vi "Convert to Array Data in Single Current Mode.vi"(7 "External\nRef":bool=TRUE, 8 "data":dbl[](array[numeric]), 9 "Electrode number, N":u16=8, 10 "Current Mode":u8[](array[numeric]), 11 "Array Mode":u16(ring) items=["None", "Gradient + Dipole dipole", "Gradient", "Dipole Dipole", "Schlumberger"]) -> (3 "String":string)   [LabVIEW 2023]
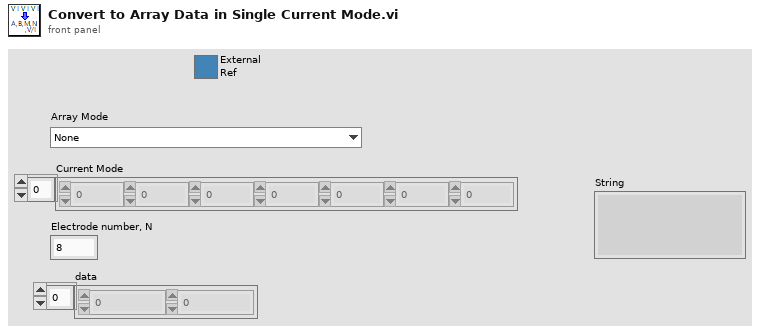
[diagram p1: front panel]
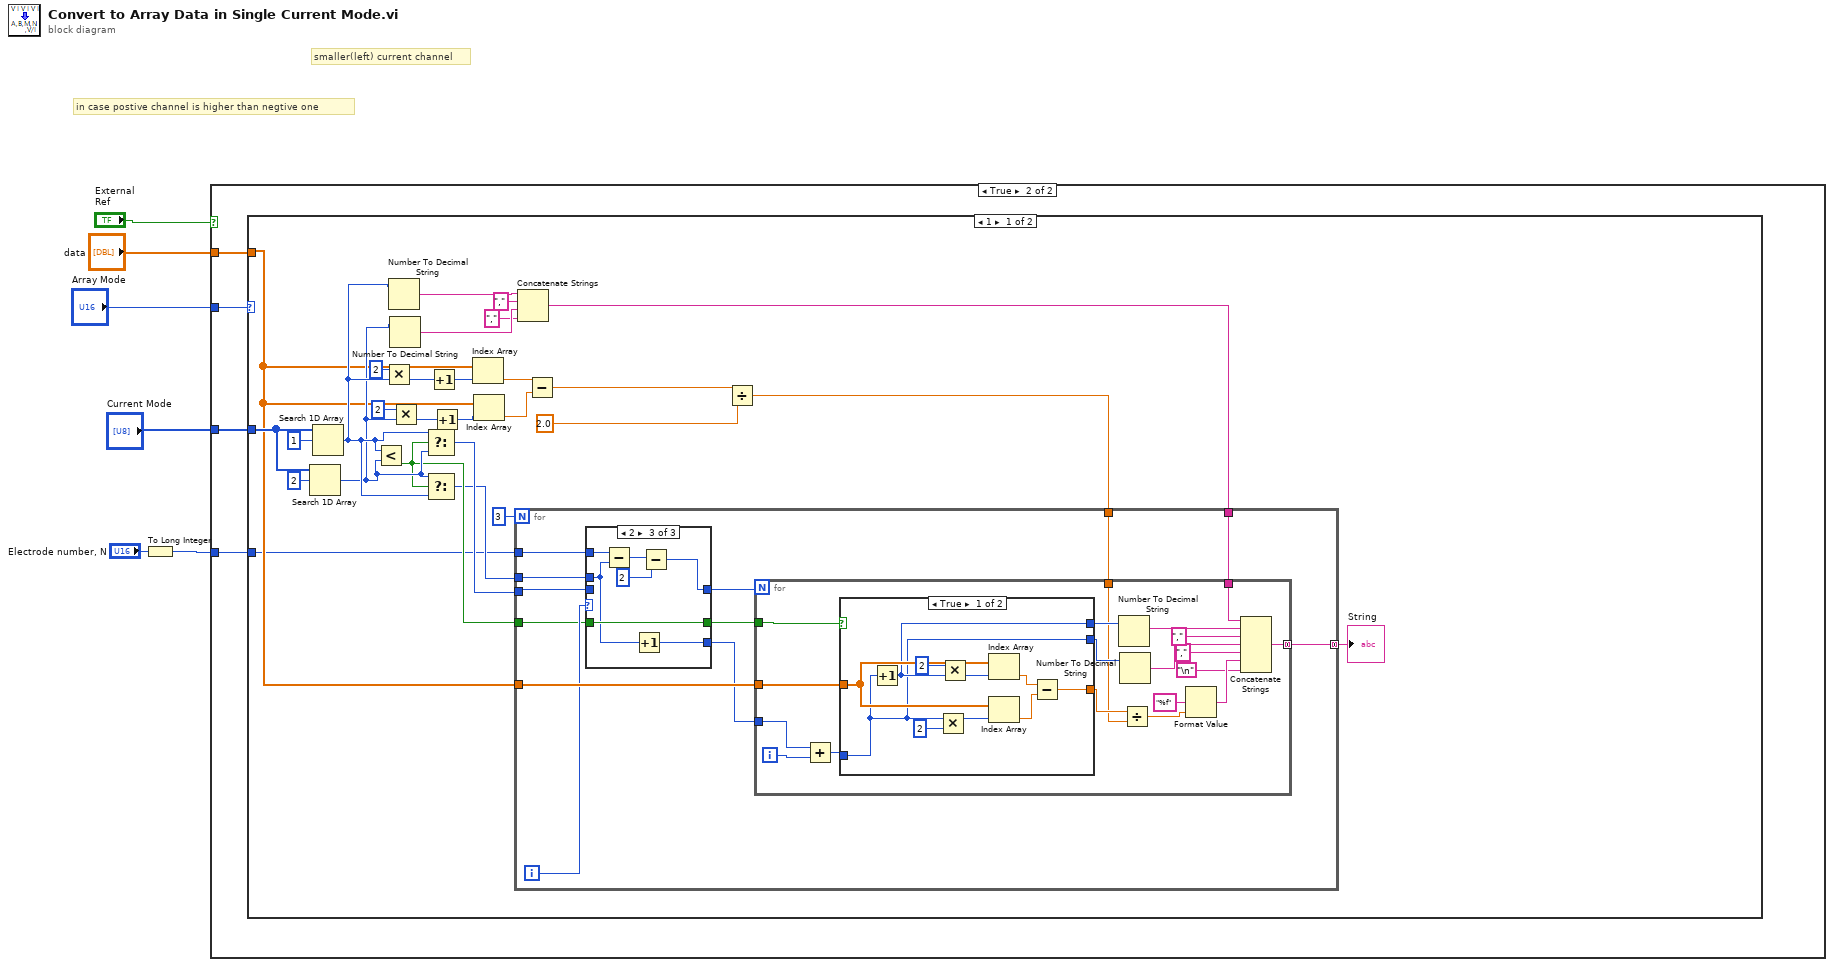
[diagram p0: block diagram]
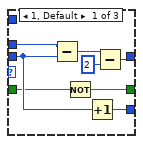
[diagram p3: hidden frame]
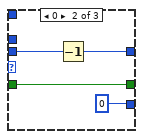
[diagram p4: hidden frame]
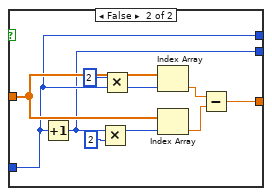
[diagram p5: hidden frame]
diagram:
  # "smaller(left) current channel"
  # "in case postive channel is higher than negtive one"
  n1 = To Long Integer(number="Electrode number, N") -> (32bit integer=w1:i32)
  n2 = case shown="True" "External\nRef" {
    tunnel: "Array Mode" -> [_ w10]
    tunnel: "Current Mode" -> [_ w9]
    tunnel: "data" -> [_ w8]
    tunnel: w1 -> [_ w7]
    frame False {
    }
    frame True {
      n3 = case shown="1" w10 {
        tunnel: w9 -> [w36 _]
        tunnel: w8 -> [w16 _]
        tunnel: w7 -> [w11 _]
        frame 1 {
          n4 = Search 1D Array(1D array=w36, element=u8 2) -> (index of element=w30:i32)  [unwired: 1 in]
          n5 = Search 1D Array(1D array=w36, element=u8 1) -> (index of element=w31:i32)  [unwired: 1 in]
          n6 = Less?(x=w31, y=w30) -> (x < y?=w19:bool)
          n7 = Multiply(x=2, y=w31) -> (x*y=w25:i32)
          n8 = Number To Decimal String(number=w31) -> (decimal integer string=w35:string)  [unwired: 1 in]
          n9 = Number To Decimal String(number=w30) -> (decimal integer string=w33:string)  [unwired: 1 in]
          n10 = Multiply(x=2, y=w30) -> (x*y=w22:i32)
          n11 = Select(t=w31, s=w19, f=w30) -> (s? t:f=w14:i32)
          n12 = Select(t=w30, s=w19, f=w31) -> (s? t:f=w13:i32)
          n13 = Increment(x=w25) -> (x+1=w23:i32)
          n14 = Increment(x=w22) -> (x+1=w20:i32)
          n15 = Index Array(array=w16, index=w23) -> (element=w29:dbl)
          n16 = Index Array(array=w16, index=w20) -> (element=w28:dbl)
          n17 = Concatenate Strings(w35, "," ("string"), w33, "," ("string")) -> (w17:string)
          n18 = Subtract(x=w29, y=w28) -> (x-y=w27:dbl)
          n19 = Divide(x=w27, y=2.0) -> (x/y=w18:dbl)
          n20 = for {
            N: 3 -> [_]
            tunnel: w19 -> [w44]
            tunnel: w18 -> [w50]
            tunnel: w17 -> [w49]
            tunnel: w16 -> [w48]
            tunnel: w14 -> [w47]
            tunnel: w13 -> [w41]
            tunnel: [w40] -> w12 mode=concatenating
            tunnel: w11 -> [w39]
            i -> [w45]
            n21 = case shown="2" w45 {
              tunnel: w47 -> [w54 w62 _]
              tunnel: [w55 w61 w65] -> w46
              tunnel: w44 -> [w52 w60 w69]
              tunnel: [w51 w60 w69] -> w43
              tunnel: [w58 0 ("s? t:f") w64] -> w42
              tunnel: w41 -> [w53 _ w63]
              tunnel: w39 -> [_ _ w68]
              frame 1, Default {
                n22 = Subtract(x=w53, y=w54) -> (x-y=w57:i32)
                n23 = Not(x=w52) -> (.not. x?=w51:bool)
                n24 = Increment(x=w54) -> (x+1=w58:i32)
                n25 = Subtract(x=w57, y=2) -> (x-y=w55:i32)
              }
              frame 0 {
                n26 = Decrement(x=w62) -> (x-1=w61:i32)
              }
              frame 2 {
                n27 = Subtract(x=w68, y=w63) -> (x-y=w67:i32)
                n28 = Increment(x=w63) -> (x+1=w64:i32)
                n29 = Subtract(x=w67, y=2) -> (x-y=w65:i32)
              }
            }
            n30 = for {
              N: w46 -> [_]
              tunnel: w43 -> [w88]
              tunnel: w48 -> [w87]
              tunnel: w49 -> [w79]
              tunnel: w50 -> [w77]
              tunnel: [w73] -> w40 mode=concatenating
              tunnel: w42 -> [w71]
              i -> [w72]
              n31 = Add(x=w71, y=w72) -> (x+y=w70:i32)
              n32 = case shown="True" w88 {
                tunnel: w87 -> [w98 w108]
                tunnel: w70 -> [w93 w104]
                tunnel: [w95 w105] -> w78
                tunnel: [w94 w104] -> w86
                tunnel: [w93 w103] -> w85
                frame True {
                  n33 = Increment(x=w93) -> (x+1=w94:i32)
                  n34 = Multiply(x=w93, y=2) -> (x*y=w90:i32)
                  n35 = Multiply(x=2, y=w94) -> (x*y=w92:i32)
                  n36 = Index Array(array=w98, index=w92) -> (element=w97:dbl)
                  n37 = Index Array(array=w98, index=w90) -> (element=w96:dbl)
                  n38 = Subtract(x=w97, y=w96) -> (x-y=w95:dbl)
                }
                frame False {
                  n39 = Increment(x=w104) -> (x+1=w103:i32)
                  n40 = Multiply(x=w103, y=2) -> (x*y=w100:i32)
                  n41 = Multiply(x=2, y=w104) -> (x*y=w102:i32)
                  n42 = Index Array(array=w108, index=w102) -> (element=w107:dbl)
                  n43 = Index Array(array=w108, index=w100) -> (element=w106:dbl)
                  n44 = Subtract(x=w107, y=w106) -> (x-y=w105:dbl)
                }
              }
              n45 = Number To Decimal String(number=w86) -> (decimal integer string=w83:string)  [unwired: 1 in]
              n46 = Number To Decimal String(number=w85) -> (decimal integer string=w81:string)  [unwired: 1 in]
              n47 = Divide(x=w78, y=w77) -> (x/y=w76:dbl)
              n48 = Format Value(format string="%f", value (0)=w76) -> (output string=w75:string)  [unwired: 1 in]
              n49 = Concatenate Strings(w79, w83, "," ("string"), w81, "," ("string"), w75, "\n") -> (w73:string)
            }
          }
          "String" <- w12
        }
        frame Default {
        }
      }
    }
  }
